vi "Test VIPB Build Job.vi"() -> ()   [LabVIEW 2014]
uses:
  Core/LabVIEW CI Service/Extensions/VIPB Build/VIPB Build/VIPB Build - STYP.ctl
  Core/LabVIEW CI Service/Classes/Status Updater/Status Updater.lvclass/Status Updater.ctl
  Core/LabVIEW CI Service/Classes/Job/Job.lvclass/Job.ctl
  Core/LabVIEW CI Service/Extensions/VIPB Build/VIPB Build/VIPB Build.lvclass
  Core/LabVIEW CI Service/Classes/Status Updater/Status Updater.lvclass
  Core/LabVIEW CI Service/Classes/Job/Job.lvclass
panel:
  in  "LabVIEW Version":string="14.0"
  in  "Install after build":bool
  in  "Workspace Path":path=path "P:/alsmith/Sales/users/ACS/LabVIEW Continuous Integration/Jenkins Sample Project/Run VI Golden DUT.vi"
  out "Results":T1 {"Status" items=["Service Error"=504, "Abort"=503, "Fail"=500, "Pass"=200]}
  out "Steps":string[](array[string])
  out "Progress Percents":u32[](array[numeric])
  in  "VI Path":path=path "P:/alsmith/Sales/users/ACS/LabVIEW Continuous Integration/Jenkins Sample Project/Run VI Golden DUT.vi"
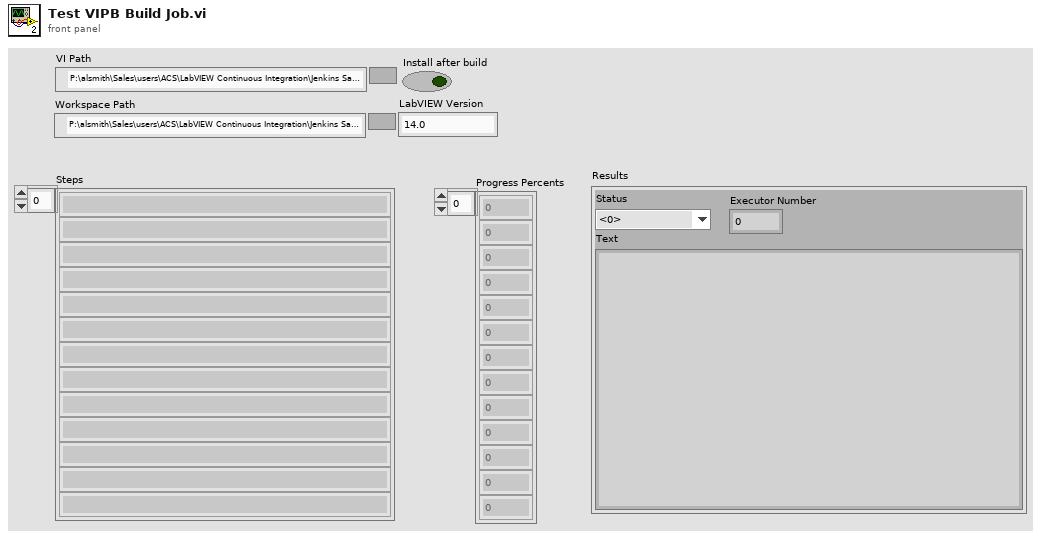
[diagram p1: front panel]
types:
  T1 = cluster{"Status":u16, "Text":string, "Executor Number":i32}
  T2 = typedef "VIPB Build - STYP.ctl" = cluster{"VIPB Path":string, "Install after build":bool, "LabVIEW Version":string}
  T3 = cluster{"Event Registration Refnum":refnum<event-registration>, "Event Registration Refnum":refnum<event-registration>}
  T4 = typedef "Job Results - STYP.ctl" = cluster{"Status":u16, "Text":string, "Executor Number":i32}
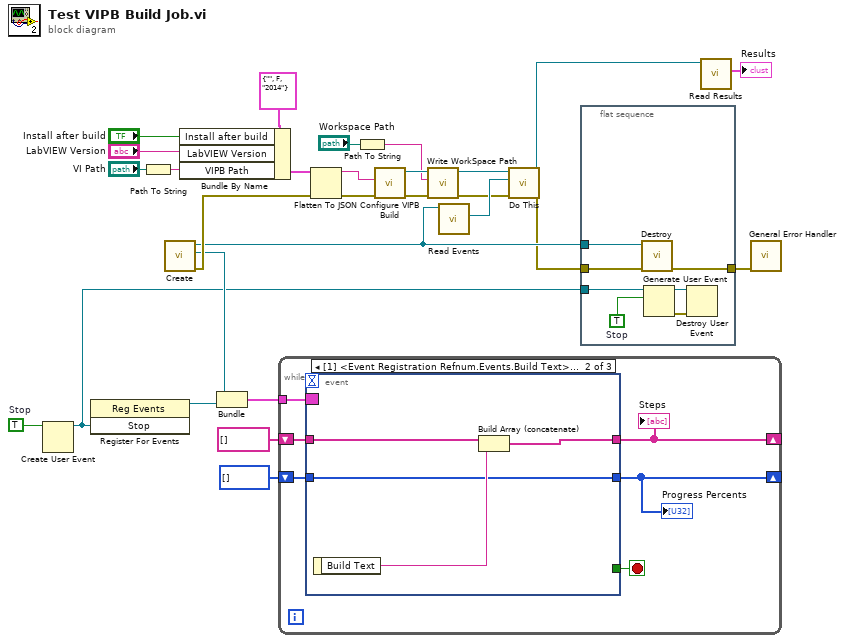
[diagram p0: block diagram]
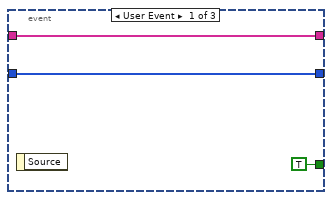
[diagram p2: hidden frame]
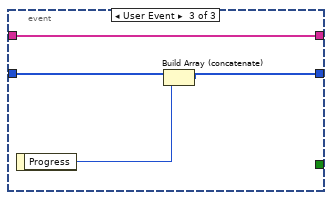
[diagram p3: hidden frame]
diagram:
  w25 = TRUE  # Stop
  n1 = Create User Event(user event datatype=w25) -> (user event=w21:refnum<user-event>)  [unwired: 1 in, 1 out]
  n2 = register-events(w21) -> (reference out=w22:refnum<event-registration>)  [unwired: 2 in, 1 out]
  n3 = Path To String(path="VI Path") -> (string=w9:string)
  n4 = call "Create.vi"() -> ("error out"=w26:errorcluster, "Event Registration Refnum"=w24:refnum<event-registration>, "Status Updater out"=w16:refnum<class "Status Updater.lvclass">)  [unwired: 9 in]
  n5 = Bundle By Name(cluster=T2 {"VIPB Path"="", "Install after build"=FALSE, "LabVIEW Version"="2014"} ("VIPB Build"), "Install after build"="Install after build", "LabVIEW Version"="LabVIEW Version", "VIPB Path"=w9) -> (w28:T2)
  n6 = Bundle("Event Registration Refnum"=w24, "Event Registration Refnum"=w22) -> (w23:T3)  [unwired: 1 in]
  n7 = while {
    tunnel: w23 -> [w34]
    shift-right: [w30] -> _
    shift-left: string[] [] -> [w32]
    shift-right: [w29] -> _
    shift-left: u32[] [] -> [w31]
    stop <- w33 stop-if-true
    n8 = event shown="[1] <Event Registration Refnum.Events.Build Text>: User Event" {
      selector: w34 -> [_ _ _]
      dyn-events: _ -> [_ _ _]
      timeout: _ -> [_ _ _]
      tunnel: [TRUE _ _] -> w33
      tunnel: w32 -> [w36 w41 w45]
      tunnel: [w36 w40 w45] -> w30
      tunnel: w31 -> [w35 w38 w44]
      tunnel: [w35 w38 w43] -> w29
      event User Event {
        n9 = event-data() -> ()  [unwired: 1 in, 1 out]
      }
      event User Event {
        n10 = event-data() -> ("Build Text"=w39:string)  [unwired: 1 in]
        n11 = Build Array (concatenate)(w41, w39) -> (w40:string[])
      }
      event User Event {
        n12 = event-data() -> ("Progress"=w42:u32)  [unwired: 1 in]
        n13 = Build Array (concatenate)(w44, w42) -> (w43:u32[])
      }
    }
    "Steps" <- w30
    "Progress Percents" <- w29
  }
  n14 = Flatten To JSON(anything=w28, error in (no error)=w26) -> (JSON string=w14:string, 11:w15:errorcluster)  [unwired: 1 in]
  n15 = Path To String(path="Workspace Path") -> (string=w5:string)
  n16 = call "Configure VIPB Build.vi"("error in (no error)"=w15, "JSON string"=w14) -> ("error out"=w6:errorcluster, "VIPB Build out"=w7:refnum<class "VIPB Build.lvclass">)  [unwired: 8 in]
  n17 = call "Write WorkSpace Path.vi"("error in (no error)"=w6, "WorkSpace Path"=w5, "Job in"=w7) -> ("error out"=w3:errorcluster, "Job out"=w4:refnum<class "VIPB Build.lvclass">)  [unwired: 7 in]
  n18 = call "Read Events.vi"("Status Updater in"=w16) -> ("Status Events"=w12:refnum<class "Status Events.lvclass">)  [unwired: 10 in]
  n19 = call-dynamic "Do This.vi"("error in (no error)"=w3, "Status Events"=w12, "VIPB Build in"=w4) -> ("error out"=w10:errorcluster, "VIPB Build out"=w11:refnum<class "VIPB Build.lvclass">)  [unwired: 7 in]
  n20 = flat-sequence {
    tunnel: w16 -> [w52]
    tunnel: w10 -> [w51]
    tunnel: w21 -> [w49]
    tunnel: [w48] -> w18
    frame #0 {
      w50 = TRUE  # Stop
      n21 = call "Destroy.vi"("error in (no error)"=w51, "Status Updater in"=w52) -> ("error out"=w48:errorcluster)  [unwired: 9 in]
      n22 = Generate User Event(user event=w49, event data cluster=w50) -> (user event out=w46:refnum<user-event>, error out=w47:errorcluster)  [unwired: 2 in]
      n23 = Destroy User Event(user event=w46, error in=w47) -> ()  [unwired: 1 out]
    }
  }
  n24 = call "Read Results.vi"("Job in"=w11) -> ("Results"=→"Results":T4)  [unwired: 10 in]
  n25 = call <vilib>:"General Error Handler.vi"("error in (no error)"=w18) -> ()  [unwired: 10 in, 5 out]
